vi "Cont Acq - Ch Expansion Sync - External Trigger.vi"() -> ()   [LabVIEW 2026]
uses:
  <vilib>/DAQmx/read.llb/DAQmx Read (Analog 1D Wfm NChan NSamp).vi
  <vilib>/FPGAPlugInAG/PXIe-7856R/niLvFpga_Open_PXIe-7856R.vi
  <vilib>/rvi/interface/common/dynamic/niFpgaDynamicAddResources.vi
  <vilib>/Utility/error.llb/Error Cluster From Error Code.vi
  <vilib>/rvi/errors/niLvFpgaAdjustHostInterfaceError.vi
  <vilib>/FPGAPlugInAG/Dynamic/niLvFpga_Run_Dynamic.vi
  <vilib>/DAQmx/create/channels.llb/DAQmx Create Channel (AI-Voltage-Basic).vi
  <vilib>/DAQmx/configure/timing.llb/DAQmx Timing (Sample Clock).vi
  <vilib>/DAQmx/configure/trigger.llb/DAQmx Start Trigger (Digital Edge).vi
  <vilib>/DAQmx/miscellaneous.llb/DAQmx Fill In Error Info.vi
  <vilib>/FPGAPlugInAG/Dynamic/niLvFpga_Close_Dynamic.vi
  <vilib>/rvi/interface/nirviOpenFPGA/nirviOpenFPGA.xnode
  FPGA Bitfiles/PulseAndTriggerGeneration.lvbitx
  FPGA/Pulse and Trigger Generation.vi
  <vilib>/rvi/interface/nirviReadWriteControl/nirviReadWriteControl.xnode
  <vilib>/rvi/interface/nirviMethod/nirviMethod.xnode
  <vilib>/rvi/interface/nirviCloseFPGA/nirviCloseFPGA.xnode
  <vilib>/rvi/interface/Simulation/niFpgaSimulationCallBeginRW.vi
  NiFpgaLv.dll
panel:
  out "Time Offset (secs)":dbl format="%#_p"
  out "Sample Offset":dbl
  in  "stop":bool
  out "Waveform Graph":waveform(dbl)[](graph)
  out "error out":errorcluster
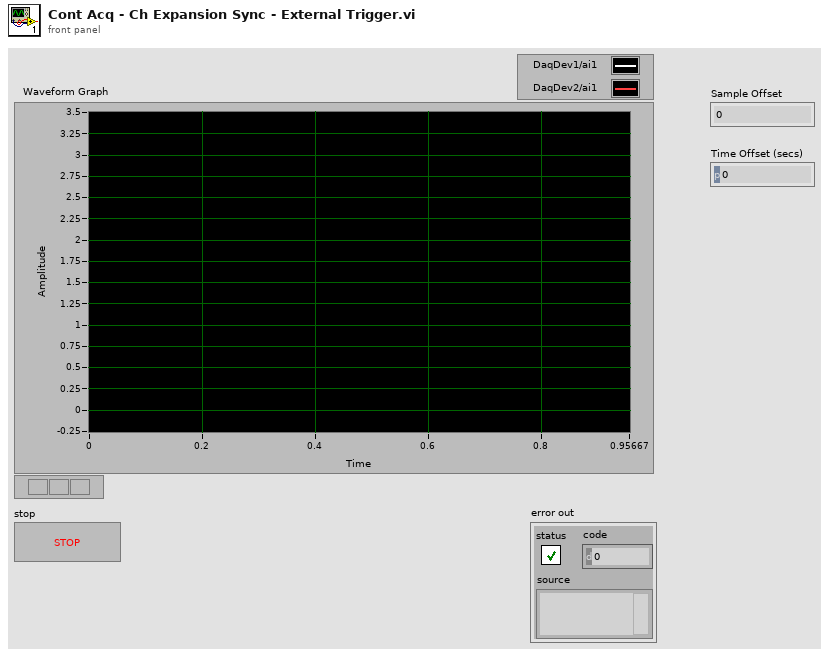
[diagram p1: front panel]
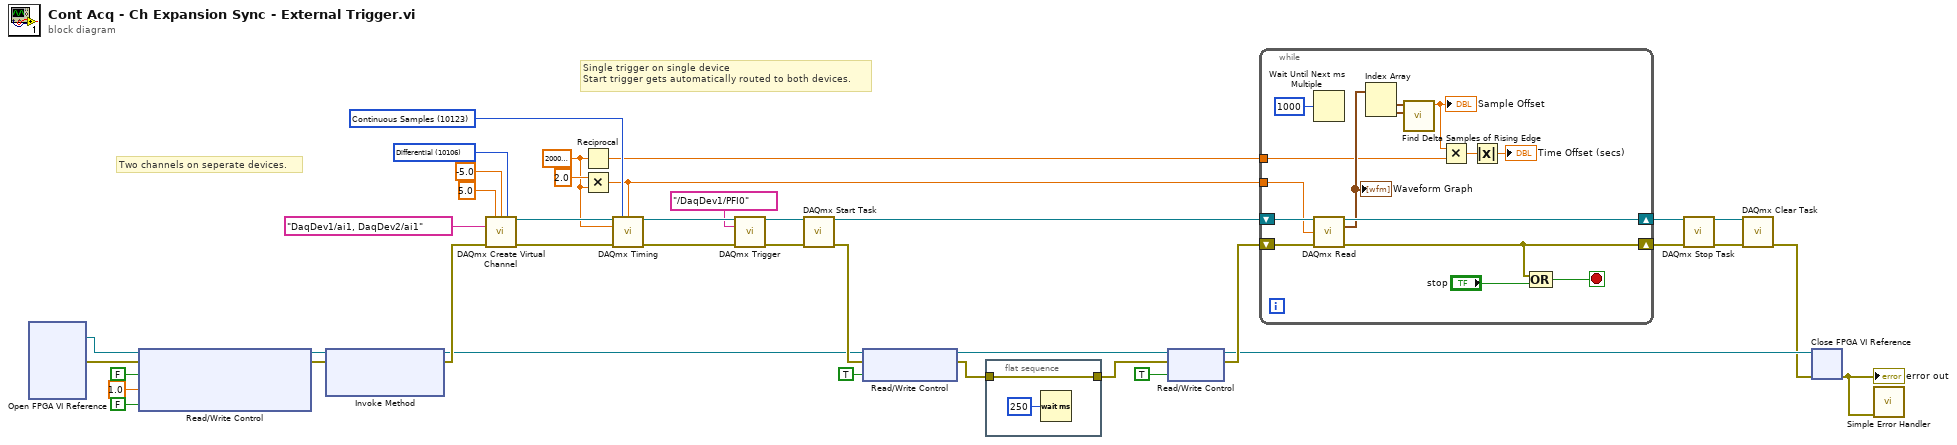
[diagram p0: block diagram]
diagram:
  w3 = 2000000.0 ("rate")
  w34 = 10123 items=["Finite Samples"=10178, "Continuous Samples"=10123, "Hardware Timed Single Point"=12522] ("sample mode")
  w39 = 10106 items=["Default"=-1, "RSE"=10083, "NRSE"=10078, "Differential"=10106, "Pseudodifferential"=12529] ("input terminal configuration")
  # "Single trigger on single device\nStart trigger gets automatically routed to both devices."
  # "Two channels on seperate devices."
  n1 = xnode "Open FPGA VI Reference"() -> ("FPGA VI Reference Out"=w27:refnum<k20>, "error out"=w26:errorcluster)  [unwired: 2 in]
  n2 = xnode "Read/Write Control"("FPGA VI Reference In"=w27, "error in"=w26, "Enable Output"=FALSE ("Connector1/DIO0"), "Requested Output Frequency"=sgl 1.0 ("Requested Clock frequency"), "Trigger"=FALSE) -> ("FPGA VI Reference Out"=w24:refnum<k20>, "error out"=w23:errorcluster)
  n3 = xnode "Invoke Method"("FPGA VI Reference In"=w24, "error in"=w23) -> ("FPGA VI Reference Out"=w9:refnum<k20>, "error out"=w22:errorcluster)  [unwired: 1 in]
  n4 = call-poly <vilib>:"DAQmx Create Virtual Channel.vi"("maximum value"=5.0, "minimum value"=-5.0, "input terminal configuration"=w39, "physical channels"=tag "DaqDev1/ai1, DaqDev2/ai1", "error in"=w22) -> ("task out"=w36:refnum<k21>, "error out"=w35:errorcluster)  [unwired: 9 in]
  n5 = Reciprocal(x=w3) -> (1/x=w2:dbl)
  n6 = Multiply(x=2.0, y=w3) -> (x*y=w16:dbl)
  n7 = call-poly <vilib>:"DAQmx Timing.vi"("task/channels in"=w36, "sample mode"=w34, "samples per channel"=w16, "rate"=w3, "error in"=w35) -> ("task out"=w33:refnum<k21>, "error out"=w13:errorcluster)  [unwired: 9 in]
  n8 = call-poly <vilib>:"DAQmx Trigger.vi"("task/channels in"=w33, "source"=tag "/DaqDev1/PFI0", "error in"=w13) -> ("task out"=w14:refnum<k21>, "error out"=w12:errorcluster)  [unwired: 11 in]
  n9 = call <vilib>:"DAQmx Start Task.vi"("task/channels in"=w14, "error in"=w12) -> ("task out"=w32:refnum<k21>, "error out"=w10:errorcluster)  [unwired: 12 in]
  n10 = xnode "Read/Write Control"("FPGA VI Reference In"=w9, "error in"=w10, "Enable Output"=TRUE ("Trigger")) -> ("FPGA VI Reference Out"=w8:refnum<k20>, "error out"=w6:errorcluster)
  n11 = flat-sequence {
    tunnel: [w41] -> w5
    tunnel: w6 -> [w41]
    frame #0 {
      n12 = Wait (ms)(milliseconds to wait=u32 250) -> ()  [unwired: 1 out]
    }
  }
  n13 = xnode "Read/Write Control"("FPGA VI Reference In"=w8, "error in"=w5, "Trigger"=TRUE ("Connector1/DIO0")) -> ("FPGA VI Reference Out"=w20:refnum<k20>, "error out"=w21:errorcluster)
  n14 = while {
    tunnel: w16 -> [w55]
    shift-right: [w56] -> w31
    shift-left: w32 -> [w57]
    shift-right: [w51] -> w29
    shift-left: w21 -> [w54]
    tunnel: w2 -> [w45]
    stop <- w50 stop-if-true
    n15 = Wait Until Next ms Multiple(millisecond multiple=u32 1000) -> ()  [unwired: 1 out]
    n16 = call-poly <vilib>:"DAQmx Read.vi"("task/channels in"=w57, "number of samples per channel"=w55, "error in"=w54) -> ("task out"=w56:refnum<k21>, "data"=w49:waveform(dbl)[], "error out"=w51:errorcluster)  [unwired: 10 in]
    "Waveform Graph" <- w49
    n17 = Index Array(array=w49) -> (element #1=w48:waveform(dbl), element #2=w47:waveform(dbl))  [unwired: 2 in]
    n18 = call "Find Delta Samples of Rising Edge.vi"("Channel 2"=w47, "Channel 1"=w48) -> ("Sample Offset"=w46:dbl)  [unwired: 9 in]
    "Sample Offset" <- w46
    n19 = Multiply(x=w46, y=w45) -> (x*y=w44:dbl)
    n20 = Absolute Value(x=w44) -> (abs(x)=→"Time Offset (secs)":dbl)
    n21 = Compound Arithmetic op=OR(w51, "stop") -> (w50:bool)
  }
  n22 = call <vilib>:"DAQmx Stop Task.vi"("task/channels in"=w31, "error in"=w29) -> ("task out"=w30:refnum<k21>, "error out"=w28:errorcluster)  [unwired: 12 in]
  n23 = call <vilib>:"DAQmx Clear Task.vi"("task in"=w30, "error in"=w28) -> ("error out"=w19:errorcluster)  [unwired: 13 in]
  n24 = xnode "Close FPGA VI Reference"("FPGA VI Reference In"=w20, "error in"=w19) -> ("error out"=w18:errorcluster)
  "error out" <- w18
  n25 = call <vilib>:"Simple Error Handler.vi"("error in (no error)"=w18) -> ()  [unwired: 4 in, 5 out]
